vi "GetSetFrameworkData.vi"(7 "Set (F)":bool, 11 "clFrameworkData In":T1) -> (3 "clFrameworkData Out":T1)   [LabVIEW 2014, in "TestFramework.lvlib"]
uses:
  TestFramework.lvlib
  TypeDefs/clFrameworkData.ctl
  Bus/NISTBus.lvclass
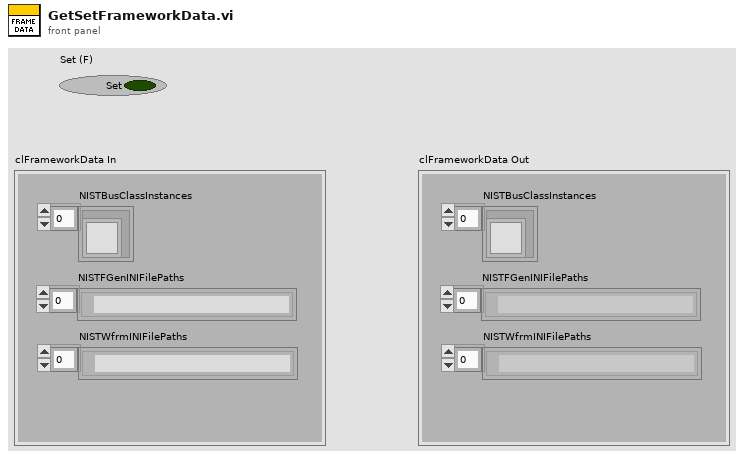
[diagram p1: front panel]
types:
  T1 = typedef "TestFramework.lvlib/clFrameworkData.ctl" = cluster{"NISTBusClassInstances":refnum<class "NISTBus.lvclass">[], "NISTFGenINIFilePaths":path[], "NISTWfrmINIFilePaths":path[]}
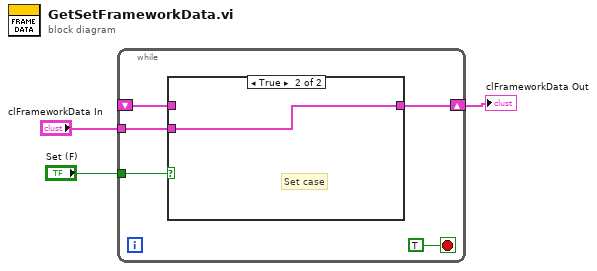
[diagram p0: block diagram]
diagram:
  n1 = while {
    tunnel: "Set (F)" -> [w7]
    tunnel: "clFrameworkData In" -> [w6]
    shift-right: [w5] -> w1
    shift-left: _ -> [w4]
    stop <- TRUE stop-if-true
    n2 = case shown="True" w7 {
      tunnel: w6 -> [_ w10]
      tunnel: [w9 w10] -> w5
      tunnel: w4 -> [w9 _]
      frame False {
        # "Get case"
      }
      frame True {
        # "Set case"
      }
    }
  }
  "clFrameworkData Out" <- w1
